vi "Time-Delayed Send Message.vi"(6 "Message Priority (Normal)":T1=enum."Normal", 7 "# Copies (0 = infinite repeat)":u32, 8 "error in (no error)":errorcluster, 9 "Milliseconds To Wait":i32=1000, 10 "Message":refnum<class "Message.lvclass">, 11 "Message Enqueuer":refnum<class "Message Enqueuer.lvclass">) -> (0 "error out":errorcluster, 2 "Delivery Notifier":refnum<notifier>)   [LabVIEW 2020]
doc: "Waits for the specified amount of time and then sends a message to an actor a specified number of times."
uses:
  <vilib>/ActorFramework/Message Enqueuer/Message Enqueuer.lvclass
  <vilib>/ActorFramework/Message/Message.lvclass
  <vilib>/ActorFramework/Time-Delayed Send Message/Time-Delay Override Options.ctl
  <vilib>/ActorFramework/Message Enqueuer/Message Priority.ctl
  <resource>/AFDebug/AF Debug.lvlib
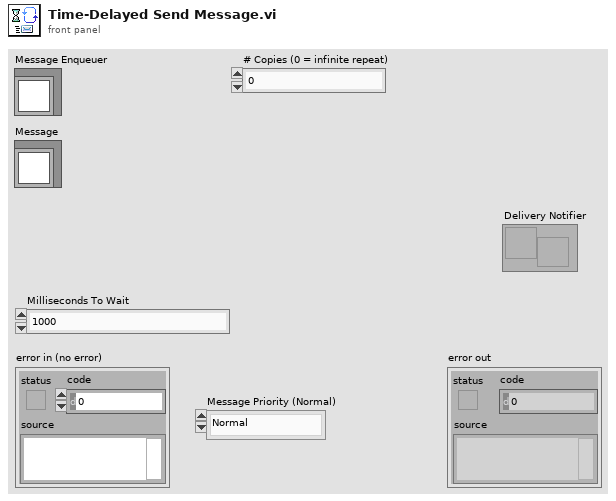
[diagram p1: front panel]
types:
  T1 = typedef "Actor Framework.lvlib/Message Enqueuer.lvclass/Message Priority.ctl" = enum16{"Low", "Normal", "High"}
  T2 = typedef "Time-Delay Override Options.ctl" = enum16{"Send next copy now", "Skip next scheduled copy", "Send next copy now and stop all further copies", "Stop all further copies"}
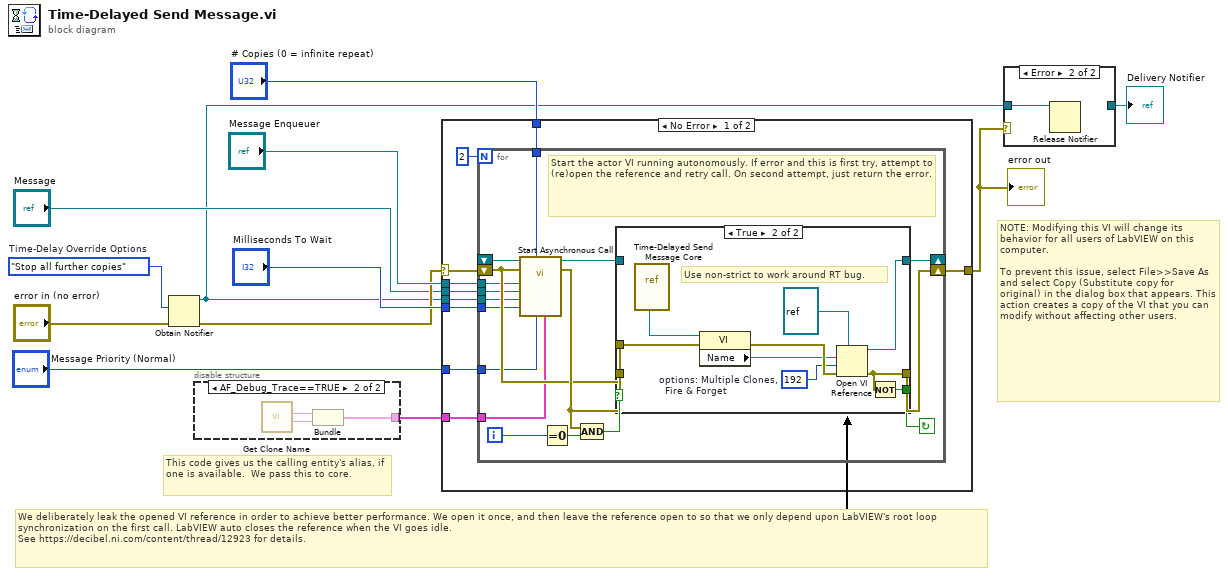
[diagram p0: block diagram]
diagram:
  w12 = Time-Delay_Override_Options."Stop all further copies"  # Time-Delay Override Options
  # "This code gives us the calling entity's alias, if one is available.  We pass this to core."
  # "We deliberately leak the opened VI reference in order to achieve better performance. We open it once, and then leave the reference open to so that we only depend upon LabVIEW's root loop synchronization on the first call. LabVIEW auto closes the reference when the VI goes idle. \nSee https://decibel.ni.com/content/thread/12923 for details."
  # "NOTE: Modifying this VI will change its behavior for all users of LabVIEW on this computer.\n\nTo prevent this issue, select File>>Save As and select Copy (Substitute copy for original) in the dialog box that appears. This action creates a copy of the VI that you can modify without affecting other users."
  n1 = Obtain Notifier(notification data type=w12, error in (no error)="error in (no error)") -> (notifier out=w2:refnum<notifier>, error out=w4:errorcluster)  [unwired: 2 in, 1 out]
  n2 = disable-structure shown="AF_Debug_Trace==TRUE" {
    disable-tunnel: [_ w13] -> w1
    frame condition #0 (active) {
    }
    frame condition #1 {
      n3 = call <resource>:"Get Clone Name.vi"() -> ("Clone ID"=w14:string, "Clone Type"=w15:string)  [unwired: 10 in]
      n4 = Bundle("Clone Type"=w15, "Clone ID"=w14) -> (w13:cluster{"Clone Type":string, "Clone ID":string})  [unwired: 1 in]
    }
  }
  n5 = case shown="No Error" w4 {
    selector: w4 -> [w23 w54]
    tunnel: [w24 w54] -> w5
    tunnel: "Message Priority (Normal)" -> [w22 _]
    tunnel: "Milliseconds To Wait" -> [w21 _]
    tunnel: "Message" -> [w20 _]
    tunnel: w2 -> [w19 _]
    tunnel: "Message Enqueuer" -> [w18 _]
    tunnel: "# Copies (0 = infinite repeat)" -> [w17 _]
    tunnel: w1 -> [w16 _]
    frame No Error {
      n6 = for {
        N: 2 -> [_]
        shift-right: [w42] -> _
        shift-left: _ -> [w34]
        shift-right: [w41] -> w24
        shift-left: w23 -> [w35]
        tunnel: w22 -> [w32]
        tunnel: w21 -> [w31]
        tunnel: w20 -> [w30]
        tunnel: w19 -> [w29]
        tunnel: w18 -> [w28]
        tunnel: w17 -> [w27]
        tunnel: w16 -> [w26]
        i -> [w38]
        stop <- w36 continue-if-true
        # "Start the actor VI running autonomously. If error and this is first try, attempt to (re)open the reference and retry call. On second attempt, just return the error."
        n7 = call-by-ref "Start Asynchronous Call"(reference=w34, error in=w35, "Trace Info"=w26, "Message Priority (Normal)"=w32, "How Many Copies (0 = infinite repeat)"=w27, "Time To Wait"=w31, "Delivery Notifier"=w29, "Message"=w30, "Message Enqueuer"=w28) -> (reference out=w33:refnum<vi>, error out=w37:errorcluster)  [unwired: 5 in]
        n8 = Equal To 0?(x=w38) -> (x = 0?=w39:bool)
        n9 = Compound Arithmetic op=AND(w37, w39) -> (w40:bool)
        n10 = case shown="True" w40 {
          tunnel: [w44 w50] -> w42
          tunnel: [w43 w48] -> w41
          tunnel: w33 -> [w44 _]
          tunnel: w37 -> [w43 _]
          tunnel: [_ w49] -> w36
          tunnel: w35 -> [_ w47]
          frame False {
          }
          frame True {
            w51 = 192  # options: Multiple Clones,   Fire & Forget
            # "Use non-strict to work around RT bug."
            n11 = vi-ref <vilib>:"Time-Delayed Send Message Core.vi"() -> (w46:refnum<vi>)
            n12 = property class="VI"(reference=w46, error in=w47) -> (error out=w53:errorcluster, "Name"=w52:string)  [unwired: 1 out]
            n13 = Open VI Reference(type specifier VI Refnum (for type only)=refnum<vi> refnum, vi path=w52, options=w51, error in (no error)=w53) -> (vi reference=w50:refnum<vi>, error out=w48:errorcluster)  [unwired: 2 in]
            n14 = Not(x=w48) -> (.not. x?=w49:bool)
          }
        }
      }
    }
    frame Error {
    }
  }
  "error out" <- w5
  n15 = case shown="Error" w5 {
    tunnel: [w55 _] -> w10
    tunnel: w2 -> [w55 w56]
    frame No Error {
    }
    frame Error {
      n16 = Release Notifier(notifier=w56) -> ()  [unwired: 2 in, 3 out]
    }
  }
  "Delivery Notifier" <- w10
